vi "Close Core.vi"(8 "Error In":errorcluster, 11 "BNT_SLMsgLogger in":refnum<class "BNT_SLMsgLogger.lvclass">) -> (0 "Error Out":errorcluster, 3 "BNT_SLMsgLogger out":refnum<class "BNT_SLMsgLogger.lvclass">)   [LabVIEW 2019, in "BNT_SLMsgLogger.lvlib" / "BNT_SLMsgLogger.lvclass"]
doc: "Close the message logger."
uses:
  BNT_SLMsgLogger.lvclass
  <vilib>/Skyline/Message/AMQP/NI Skyline Message AMQP (Sync).lvclass
  C:/Program Files (x86)/National Instruments/LabVIEW 2019/vi.lib/Skyline/Message/NI Skyline Message.lvclass
  BNT_SLMsgLogger.lvclass/BNT_SLMsgLogger.ctl
  <vilib>/Skyline/Message/NI Skyline Message.lvclass
  <vilib>/Skyline/Message/sync/NI Skyline Message Sync.lvclass
  C:/Program Files (x86)/National Instruments/LabVIEW 2019/vi.lib/Skyline/Message/sync/NI Skyline Message Sync.lvclass
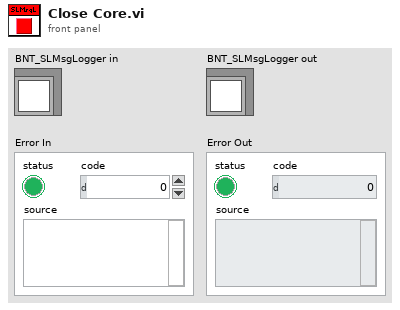
[diagram p1: front panel]
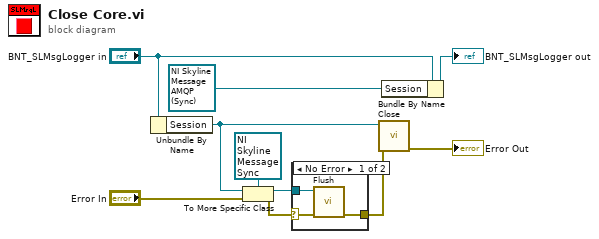
[diagram p0: block diagram]
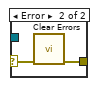
[diagram p2: hidden frame]
diagram:
  n1 = Unbundle By Name("BNT_SLMsgLogger in") -> ("Session"=w6:refnum<class "NI Skyline Message.lvclass">)
  n2 = To More Specific Class(target class=refnum<class "NI Skyline Message Sync.lvclass"> refnum ("sync message session in"), reference=w6, error in="Error In") -> (specific class reference=w4:refnum<class "NI Skyline Message Sync.lvclass">, error out=w3:errorcluster)
  n3 = case shown="No Error" w3 {
    selector: w3 -> [w12 w14]
    tunnel: w4 -> [w13 _]
    tunnel: [w11 w15] -> w1
    frame No Error {
      n4 = call-dynamic "Flush.vi"("error in (no error)"=w12, "sync message session in"=w13) -> ("error out"=w11:errorcluster)  [unwired: 8 in, 1 out]
    }
    frame Error {
      n5 = call <vilib>:"Clear Errors.vi"("error in (no error)"=w14) -> ("error out"=w15:errorcluster)  [unwired: 5 in, 1 out]
    }
  }
  n6 = call-dynamic "Close.vi"("error in (no error)"=w1, "message session"=w6) -> ("error out"=→"Error Out":errorcluster)  [unwired: 9 in]
  n7 = Bundle By Name(cluster="BNT_SLMsgLogger in", "Session"=refnum<class "NI Skyline Message AMQP (Sync).lvclass"> refnum) -> (→"BNT_SLMsgLogger out":refnum<class "BNT_SLMsgLogger.lvclass">)
